vi "Update All Values.vi"(8 "error in (no error)":errorcluster, 10 "Values":refnum<class "Type.lvclass">[](array[class]), 11 "NewEntityTemplate in":refnum<class "Test2.lvclass">) -> (0 "error out":errorcluster, 3 "NewEntityTemplate out":refnum<class "Test2.lvclass">)   [LabVIEW 2020, in "tests.lvlib" / "Test2.lvclass"]
uses:
  Test2.lvclass
  <vilib>/IlluminatedG/IG Conditum Base/Conditum/Columns/Type/Type.lvclass
  Test2.lvclass/Test2.ctl
  <vilib>/IlluminatedG/IG Conditum Base/Conditum/Columns/Integer/Integer.lvclass
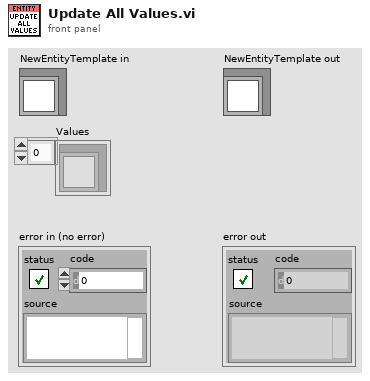
[diagram p1: front panel]
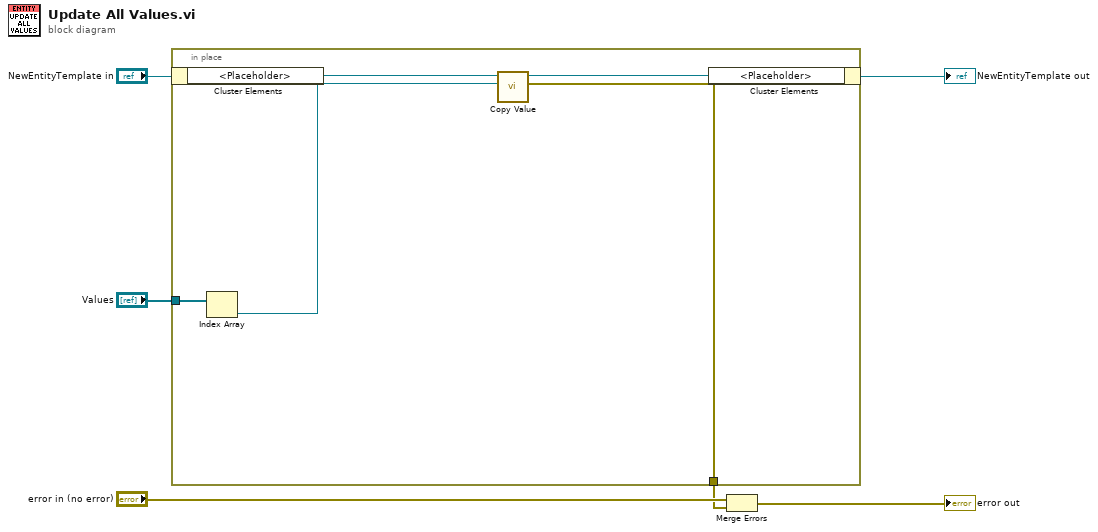
[diagram p0: block diagram]
diagram:
  n1 = in-place {
    in-place-border: "Values" -> [w10]
    in-place-border: [w8] -> w3
    n2 = in-place-cluster #1("NewEntityTemplate in") -> ("<Placeholder>"=w11:refnum<class "Integer.lvclass">)
    n3 = Index Array(array=w10) -> (element=w7:refnum<class "Type.lvclass">)  [unwired: 1 in]
    n4 = call-dynamic "Copy Value.vi"("From"=w7, "Integer in"=w11) -> ("error out"=w8:errorcluster, "Integer out"=w9:refnum<class "Integer.lvclass">)  [unwired: 8 in]
    n5 = in-place-cluster #1("<Placeholder>"=w9) -> (→"NewEntityTemplate out":refnum<class "Test2.lvclass">)
  }
  n6 = Merge Errors("error in (no error)", w3) -> (→"error out":errorcluster)
